vi "TEST - Array Size(s).vi"(8 "error in (no error)":errorcluster) -> (0 "error out":errorcluster, 2 "pass":bool)   [LabVIEW 2020, in "test_openg_variant.lvlib"]
uses:
  test_openg_variant.lvlib
  <vilib>/addons/_JKI Toolkits/Caraya/classes/Assert/Assert True.vi
  source/library/openg_variant.lvlib
  <vilib>/addons/_JKI Toolkits/Caraya/classes/Test/Test.lvclass
  <vilib>/addons/_JKI Toolkits/Caraya/classes/Assert/Assert.lvclass
panel:
  out "Failures":T1(array[cluster])
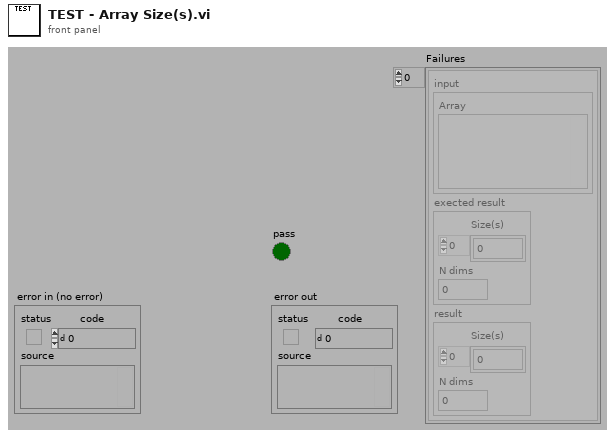
[diagram p1: front panel]
types:
  T1 = cluster{"input":cluster{"Array":variant}, "exected result":cluster{"Size(s)":u32[], "N dims":u32}, "result":cluster{"Size(s)":u32[], "N dims":u32}}[]
  T2 = cluster{"input":cluster{"Array":variant}, "exected result":cluster{"Size(s)":u32[], "N dims":u32}, "result":cluster{"Size(s)":u32[], "N dims":u32}}
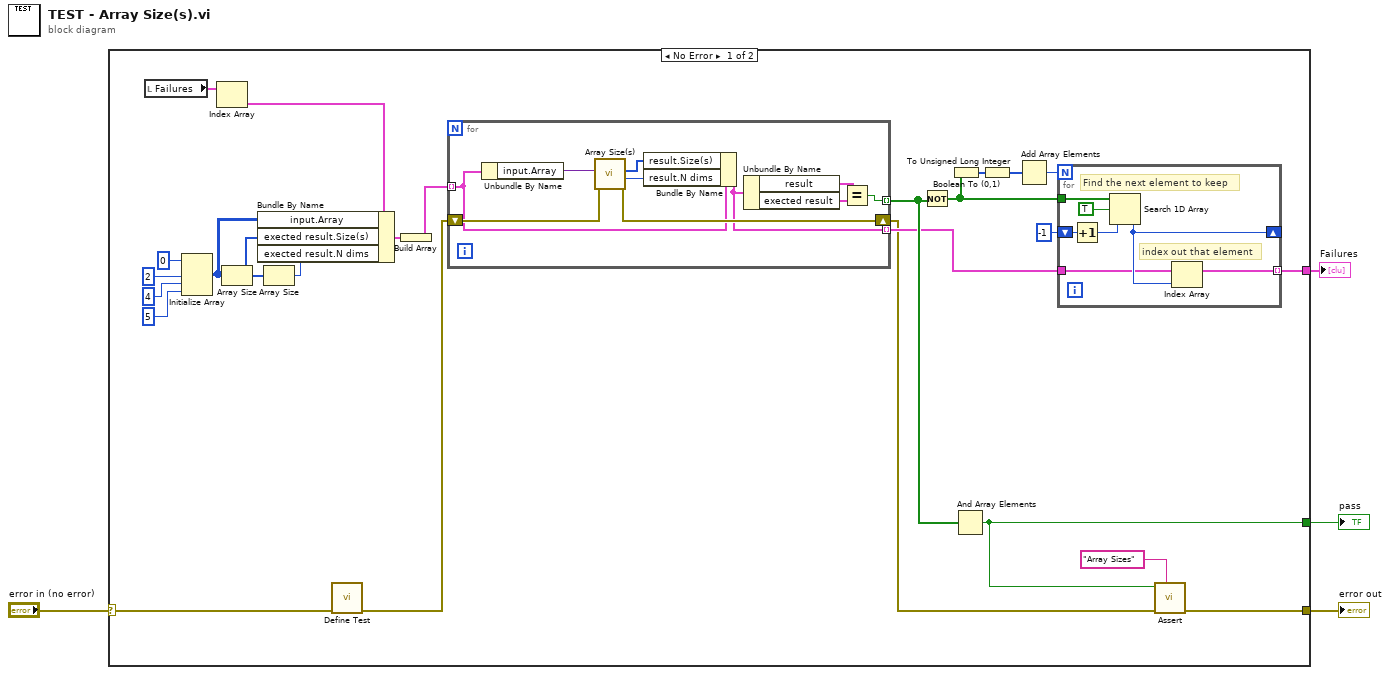
[diagram p0: block diagram]
diagram:
  n1 = case shown="No Error" "error in (no error)" {
    selector: "error in (no error)" -> [w9 w47]
    tunnel: [w5 _] -> w4
    tunnel: [w6 w47] -> w2
    tunnel: [w22 _] -> w1
    frame No Error {
      n2 = local read "Failures"() -> (w19:T1)
      n3 = Initialize Array(0, u32 2 ("Numeric"), 4 ("Numeric"), 5 ("Numeric")) -> (w11:i32[][][])
      n4 = Index Array(array=w19) -> (element=w18:T2)  [unwired: 1 in]
      n5 = Array Size(array=w11) -> (size(s)=w13:i32[])
      n6 = Array Size(array=w13) -> (size(s)=w12:i32)
      n7 = Bundle By Name(cluster=w18, "input.Array"=w11, "exected result.Size(s)"=w13, "exected result.N dims"=w12) -> (w21:T2)
      n8 = call <vilib>:"Define Test.vi"("error in (no error)"=w9) -> ("error out"=w8:errorcluster)  [unwired: 9 in, 1 out]
      n9 = Build Array(w21) -> (w20:T1)
      n10 = for {
        tunnel: w20 -> [w43] mode=indexing
        tunnel: [w46] -> w24 mode=indexing
        tunnel: [w42] -> w23 mode=indexing
        shift-right: [w44] -> w7
        shift-left: w8 -> [w45]
        n11 = Unbundle By Name(w43) -> ("input.Array"=w37:variant)
        n12 = call "Array Size(s).vi"("error in (no error)"=w45, "Array"=w37) -> ("error out"=w44:errorcluster, "N dims"=w39:u32, "Size(s)"=w40:u32[])  [unwired: 7 in]
        n13 = Bundle By Name(cluster=w43, "result.Size(s)"=w40, "result.N dims"=w39) -> (w42:T2)
        n14 = Unbundle By Name(w42) -> ("result"=w41:cluster{"Size(s)":u32[], "N dims":u32}, "exected result"=w38:cluster{"Size(s)":u32[], "N dims":u32})
        n15 = Equal?(x=w41, y=w38) -> (x = y?=w46:bool)
      }
      n16 = Not(x=w24) -> (.not. x?=w26:bool[])
      n17 = Boolean To (0,1)(Boolean=w26) -> (0, 1=w27:i16[])
      n18 = And Array Elements(Boolean array=w24) -> (logical AND=w5:bool)
      n19 = To Unsigned Long Integer(number=w27) -> (unsigned 32bit integer=w25:u32[])
      n20 = Add Array Elements(numeric array=w25) -> (sum=w28:u32)
      n21 = for {
        N: w28 -> [_]
        tunnel: w23 -> [w32]
        tunnel: w26 -> [w36]
        shift-right: [w33] -> _
        shift-left: -1 ("start index (0)") -> [w34]
        tunnel: [w31] -> w22 mode=indexing
        # "index out that element"
        # "Find the next element to keep"
        n22 = Increment(x=w34) -> (x+1=w30:i32)
        n23 = Search 1D Array(1D array=w36, element=TRUE, start index (0)=w30) -> (index of element=w33:i32)
        n24 = Index Array(array=w32, index=w33) -> (element=w31:T2)
      }
      n25 = call-poly <vilib>:"Assert.vi"("Label"="Array Sizes" ("Label (VI Title)"), "error in (no error)"=w7, "True?"=w5) -> ("error out"=w6:errorcluster)  [unwired: 7 in, 1 out]
    }
    frame Error {
    }
  }
  "pass" <- w4
  "error out" <- w2
  "Failures" <- w1
